vi "DeStringQueue.vi"(8 "error in":errorcluster, 11 "QueueIn":variant) -> (0 "error out":errorcluster, 1 "StringOut":string, 3 "QueueOut":variant)   [LabVIEW 2013]
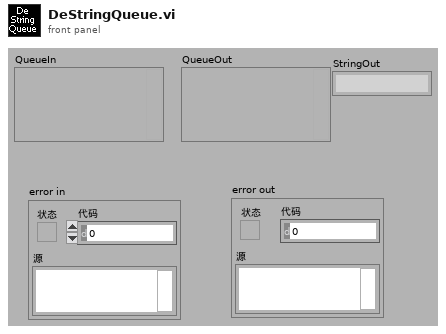
[diagram p1: front panel]
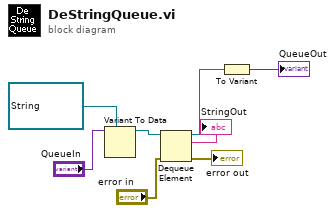
[diagram p0: block diagram]
diagram:
  n1 = Variant To Data(type=refnum<queue> refnum ("队列输出"), Variant="QueueIn") -> (data=w3:refnum<queue>)  [unwired: 1 in, 1 out]
  n2 = Dequeue Element(queue=w3, error in (no error)="error in") -> (queue out=w5:refnum<queue>, element=→"StringOut":string, error out=→"error out":errorcluster)  [unwired: 2 out]
  n3 = To Variant(anything=w5) -> (Variant=→"QueueOut":variant)
